vi "Stop Core.vi"(10 "final error code":i32, 11 "CS++IEFWerner in":refnum<class "CS++IEFWerner.lvclass">) -> (3 "CS++IEFWerner out":refnum<class "CS++IEFWerner.lvclass">)   [LabVIEW 2015, in "CS++IEFWerner.lvlib" / "CS++IEFWerner.lvclass"]
doc: "(<B>Filename</B>: Actor Framework.lvlib:Actor.lvclass:Stop Core.vi)\n\nDefines what the actor does before it stops. Use the <B>final error code</B> input to determine whether the actor shut down in response to an error.\n\nBy default, this method does nothing. A descendant class may override it to define behavior, such as shutting down any processes the actor initiated in its override of the Actor Core method."
uses:
  CS++IEFWerner.lvclass
  CS++IEFWerner.lvclass/CS++IEFWerner.ctl
  CSPP_DeviceBase/CS++Motor/CS++Motor.lvclass
  CSPP_Core/Classes/CS++ProcessVariables/PVConnection/PVConnection.lvclass
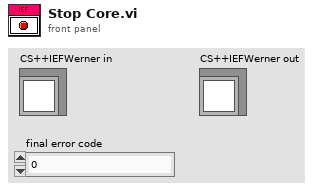
[diagram p1: front panel]
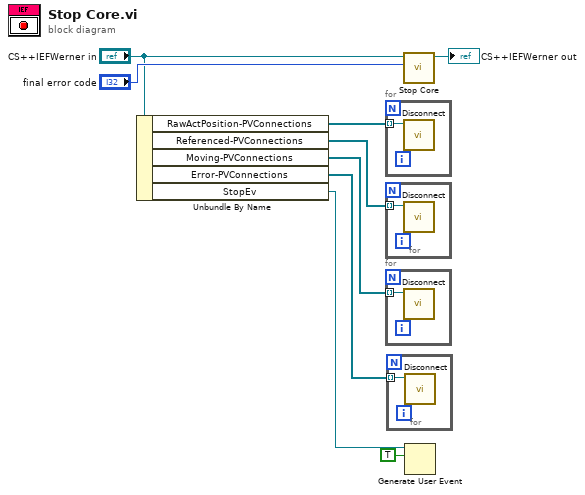
[diagram p0: block diagram]
diagram:
  n1 = Unbundle By Name("CS++IEFWerner in") -> ("RawActPosition-PVConnections"=w7:refnum<class "PVConnection.lvclass">[], "Referenced-PVConnections"=w6:refnum<class "PVConnection.lvclass">[], "Moving-PVConnections"=w5:refnum<class "PVConnection.lvclass">[], "Error-PVConnections"=w4:refnum<class "PVConnection.lvclass">[], "StopEv"=w2:refnum<user-event>)
  n2 = for {
    tunnel: w7 -> [w10] mode=indexing
    n3 = call "Disconnect.vi"("PVConnection in"=w10) -> ()  [unwired: 9 in, 2 out]
  }
  n4 = for {
    tunnel: w6 -> [w11] mode=indexing
    n5 = call "Disconnect.vi"("PVConnection in"=w11) -> ()  [unwired: 9 in, 2 out]
  }
  n6 = for {
    tunnel: w5 -> [w12] mode=indexing
    n7 = call "Disconnect.vi"("PVConnection in"=w12) -> ()  [unwired: 9 in, 2 out]
  }
  n8 = for {
    tunnel: w4 -> [w13] mode=indexing
    n9 = call "Disconnect.vi"("PVConnection in"=w13) -> ()  [unwired: 9 in, 2 out]
  }
  n10 = call-parent "Stop Core.vi"("final error code"="final error code", "CS++Motor in"="CS++IEFWerner in") -> ("CS++Motor out"=→"CS++IEFWerner out":refnum<class "CS++IEFWerner.lvclass">)  [unwired: 9 in]
  n11 = Generate User Event(user event=w2, event data cluster=TRUE ("event data")) -> ()  [unwired: 2 in, 2 out]
